vi "Stop Watch.vi"(8 "error In":errorcluster, 9 "Time Stamp Select In":T1, 11 "Stop Wtch ID (0-29) In":i32=-1) -> (0 "error Out":errorcluster, 2 "Time (S) Out":dbl, 3 "ID Out":i32)   [LabVIEW 2015]
uses:
  TypeDefs_Utility/ENUM_Time_Type Select.ctl
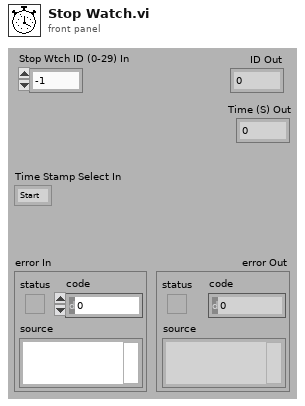
[diagram p1: front panel]
types:
  T1 = typedef "ENUM_Time_Type Select.ctl" = enum16{"Start", "Time", "Cycle"}
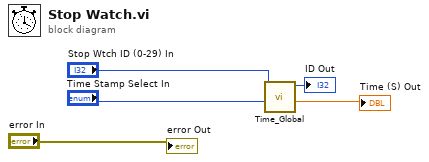
[diagram p0: block diagram]
diagram:
  n1 = call "Time_Global.vi"("Time Stamp Select"="Time Stamp Select In", "ID"="Stop Wtch ID (0-29) In") -> ("Time (S)"=→"Time (S) Out":dbl, "ID Out"=→"ID Out":i32)  [unwired: 8 in]
  "error Out" <- "error In"
